vi "NEW RW Controls INI.vi"(1 "Filepath":path, 2 "Read (F)":bool, 7 "ControlArray In":T1(array[cluster]), 11 "Error In":errorcluster) -> (8 "ControlArray Out":T1(array[cluster]), 15 "Error Out":errorcluster)   [LabVIEW 2013]
uses:
  <vilib>/Utility/config.llb/Read Key (Double).vi
  <vilib>/Utility/config.llb/Write Key (Double).vi
  <vilib>/Utility/config.llb/NI_LVConfig.lvlib
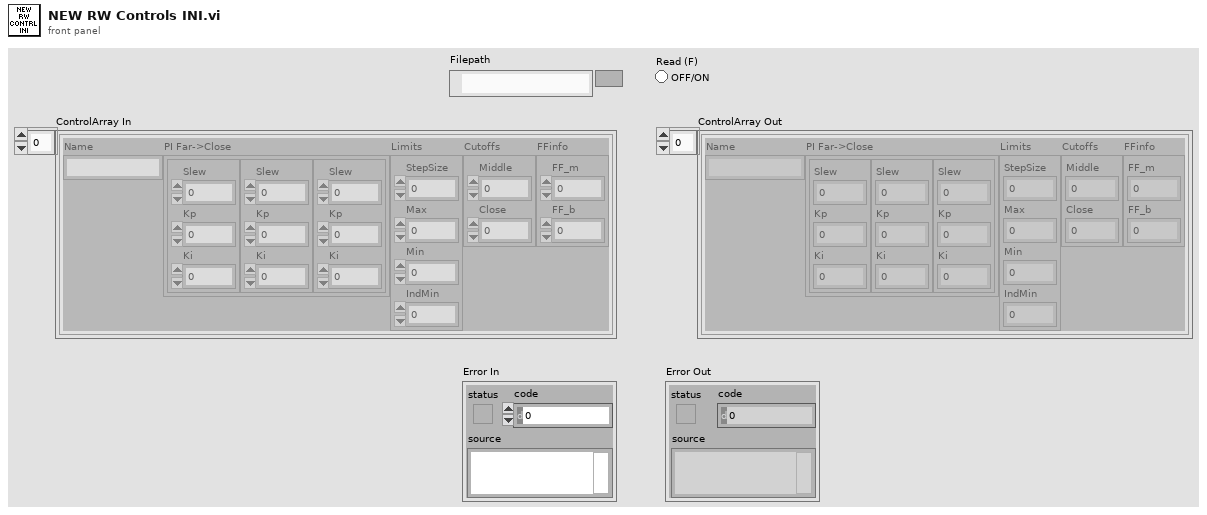
[diagram p1: front panel]
types:
  T1 = cluster{"Name":string, "PI Far->Close":cluster{"Slew":dbl, "Kp":dbl, "Ki":dbl}[], "Limits":cluster{"StepSize":dbl, "Max":dbl, "Min":dbl, "IndMin":dbl}, "Cutoffs":cluster{"Middle":dbl, "Close":dbl}, "FFinfo":cluster{"FF_m":dbl, "FF_b":dbl}}[]
  T2 = typedef "NI_LVConfig.lvlib/Config Data RefNum.ctl" = refnum<k1>
  T3 = cluster{"StepSize":dbl, "Max":dbl, "Min":dbl, "IndMin":dbl}
  T4 = cluster{"value":dbl, "value":dbl, "value":dbl, "value":dbl}
  T5 = cluster{"Name":string, "PI Far->Close":cluster{"Slew":dbl, "Kp":dbl, "Ki":dbl}[], "Limits":cluster{"StepSize":dbl, "Max":dbl, "Min":dbl, "IndMin":dbl}, "Cutoffs":cluster{"Middle":dbl, "Close":dbl}, "FFinfo":cluster{"FF_m":dbl, "FF_b":dbl}}
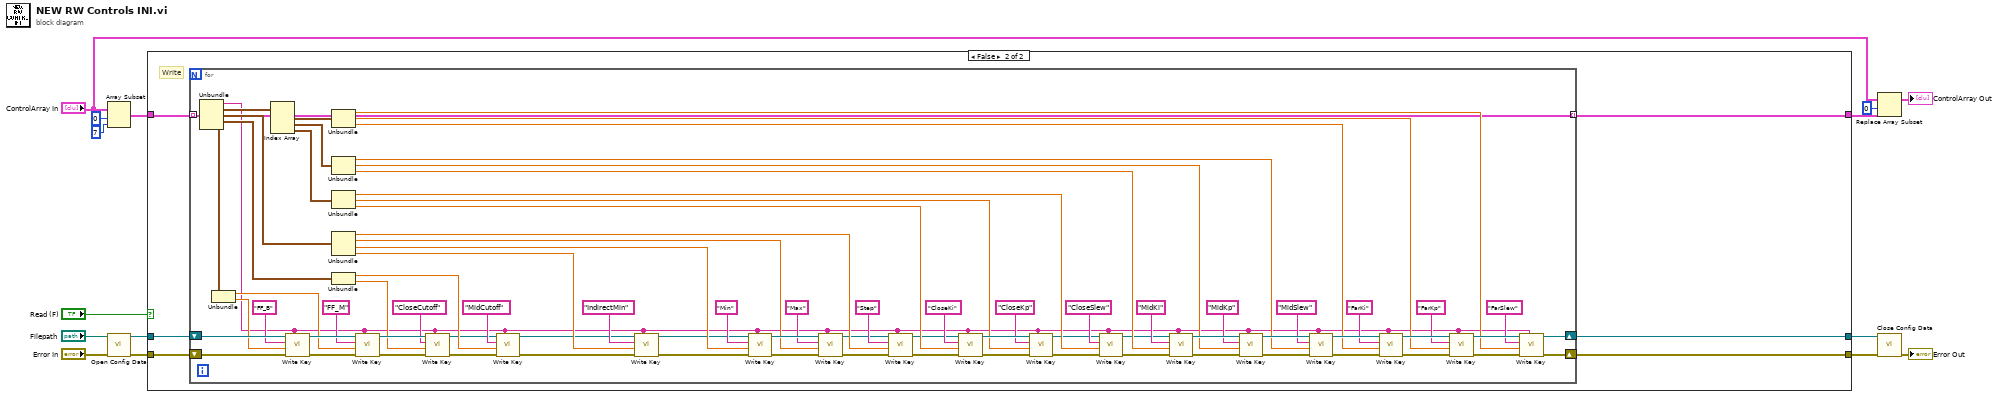
[diagram p0: block diagram]
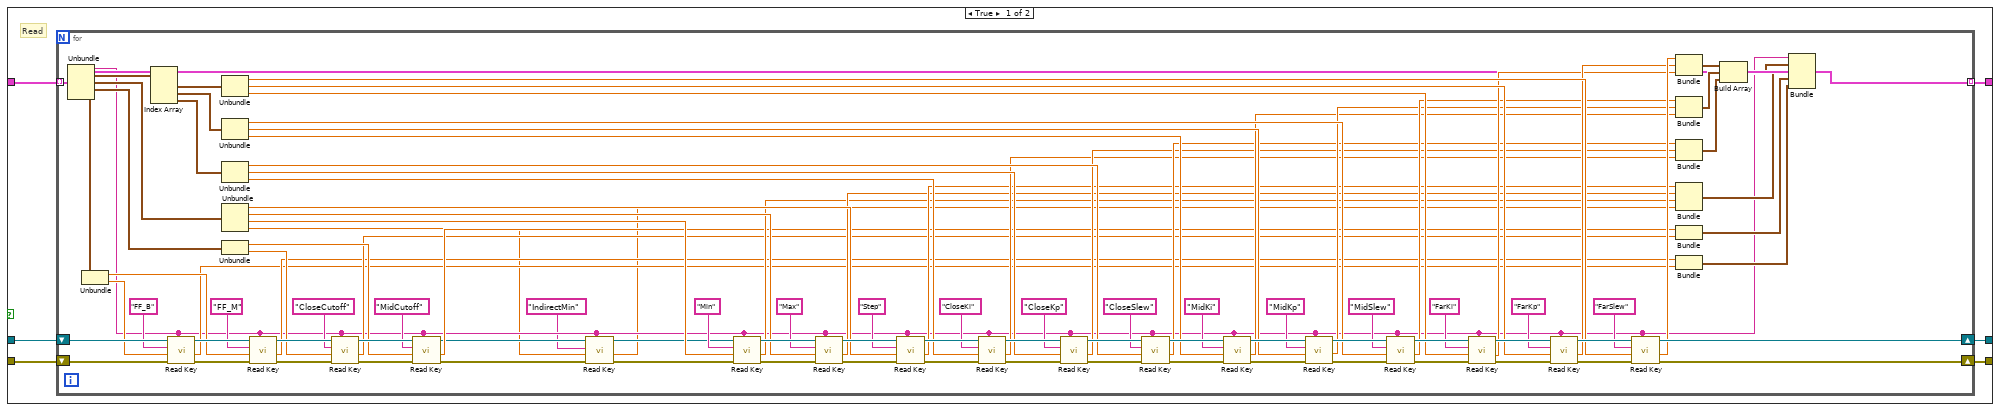
[diagram p2: hidden frame]
diagram:
  n1 = Array Subset(array="ControlArray In", index=0, length=7) -> (w1:T1)
  n2 = call <vilib>:"Open Config Data.vi"("error in (no error)"="Error In", "configuration file path"="Filepath") -> ("error out"=w11:errorcluster, "refnum"=w10:T2)  [unwired: 7 in, 1 out]
  n3 = case shown="False" "Read (F)" {
    tunnel: w11 -> [w17 w131]
    tunnel: w10 -> [w18 w130]
    tunnel: w1 -> [w21 w129]
    tunnel: [w20 w128] -> w9
    tunnel: [w19 w127] -> w8
    tunnel: [w16 w126] -> w5
    frame True {
      # "Read"
      n4 = for {
        tunnel: w21 -> [w35] mode=indexing
        shift-right: [w89] -> w19
        shift-left: w18 -> [w87]
        shift-right: [w90] -> w20
        shift-left: w17 -> [w88]
        tunnel: [w30] -> w16 mode=indexing
        n5 = Unbundle(w35) -> ("Name"=w28:string, "PI Far->Close"=w125:cluster{"Slew":dbl, "Kp":dbl, "Ki":dbl}[], "Limits"=w122:T3, "Cutoffs"=w123:cluster{"Middle":dbl, "Close":dbl}, "FFinfo"=w124:cluster{"FF_m":dbl, "FF_b":dbl})
        n6 = Unbundle(w124) -> ("FF_m"=w69:dbl, "FF_b"=w86:dbl)
        n7 = Index Array(array=w125) -> (element #1=w119:cluster{"Slew":dbl, "Kp":dbl, "Ki":dbl}, element #2=w120:cluster{"Slew":dbl, "Kp":dbl, "Ki":dbl}, element #3=w121:cluster{"Slew":dbl, "Kp":dbl, "Ki":dbl})  [unwired: 3 in]
        n8 = call-poly <vilib>:"Read Key.vi"("section"=w28, "error in (no error)"=w88, "default value"=w86, "key"="FF_B", "refnum"=w87) -> ("error out"=w117:errorcluster, "value"=w39:dbl, "refnum out"=w118:T2)  [unwired: 3 in, 1 out]
        n9 = Unbundle(w119) -> ("Slew"=w55:dbl, "Kp"=w56:dbl, "Ki"=w57:dbl)
        n10 = Unbundle(w120) -> ("Slew"=w58:dbl, "Kp"=w59:dbl, "Ki"=w60:dbl)
        n11 = Unbundle(w121) -> ("Slew"=w61:dbl, "Kp"=w62:dbl, "Ki"=w63:dbl)
        n12 = Unbundle(w122) -> ("StepSize"=w64:dbl, "Max"=w65:dbl, "Min"=w66:dbl, "IndMin"=w24:dbl)
        n13 = Unbundle(w123) -> ("Middle"=w67:dbl, "Close"=w68:dbl)
        n14 = call-poly <vilib>:"Read Key.vi"("section"=w28, "error in (no error)"=w117, "default value"=w69, "key"="FF_M", "refnum"=w118) -> ("error out"=w116:errorcluster, "value"=w40:dbl, "refnum out"=w115:T2)  [unwired: 3 in, 1 out]
        n15 = call-poly <vilib>:"Read Key.vi"("section"=w28, "error in (no error)"=w116, "default value"=w68, "key"="CloseCutoff", "refnum"=w115) -> ("error out"=w113:errorcluster, "value"=w41:dbl, "refnum out"=w114:T2)  [unwired: 3 in, 1 out]
        n16 = call-poly <vilib>:"Read Key.vi"("section"=w28, "error in (no error)"=w113, "default value"=w67, "key"="MidCutoff", "refnum"=w114) -> ("error out"=w26:errorcluster, "value"=w42:dbl, "refnum out"=w29:T2)  [unwired: 3 in, 1 out]
        n17 = call-poly <vilib>:"Read Key.vi"("section"=w28, "error in (no error)"=w26, "default value"=w24, "key"="IndirectMin", "refnum"=w29) -> ("error out"=w25:errorcluster, "value"=w23:dbl, "refnum out"=w27:T2)  [unwired: 3 in, 1 out]
        n18 = call-poly <vilib>:"Read Key.vi"("section"=w28, "error in (no error)"=w25, "default value"=w66, "key"="Min", "refnum"=w27) -> ("error out"=w112:errorcluster, "value"=w43:dbl, "refnum out"=w105:T2)  [unwired: 3 in, 1 out]
        n19 = call-poly <vilib>:"Read Key.vi"("section"=w28, "error in (no error)"=w112, "default value"=w65, "key"="Max", "refnum"=w105) -> ("error out"=w111:errorcluster, "value"=w44:dbl, "refnum out"=w104:T2)  [unwired: 3 in, 1 out]
        n20 = call-poly <vilib>:"Read Key.vi"("section"=w28, "error in (no error)"=w111, "default value"=w64, "key"="Step", "refnum"=w104) -> ("error out"=w110:errorcluster, "value"=w45:dbl, "refnum out"=w103:T2)  [unwired: 3 in, 1 out]
        n21 = call-poly <vilib>:"Read Key.vi"("section"=w28, "error in (no error)"=w110, "default value"=w63, "key"="CloseKi", "refnum"=w103) -> ("error out"=w109:errorcluster, "value"=w46:dbl, "refnum out"=w102:T2)  [unwired: 3 in, 1 out]
        n22 = call-poly <vilib>:"Read Key.vi"("section"=w28, "error in (no error)"=w109, "default value"=w62, "key"="CloseKp", "refnum"=w102) -> ("error out"=w108:errorcluster, "value"=w47:dbl, "refnum out"=w101:T2)  [unwired: 3 in, 1 out]
        n23 = call-poly <vilib>:"Read Key.vi"("section"=w28, "error in (no error)"=w108, "default value"=w61, "key"="CloseSlew", "refnum"=w101) -> ("error out"=w107:errorcluster, "value"=w48:dbl, "refnum out"=w100:T2)  [unwired: 3 in, 1 out]
        n24 = call-poly <vilib>:"Read Key.vi"("section"=w28, "error in (no error)"=w107, "default value"=w60, "key"="MidKi", "refnum"=w100) -> ("error out"=w106:errorcluster, "value"=w49:dbl, "refnum out"=w99:T2)  [unwired: 3 in, 1 out]
        n25 = call-poly <vilib>:"Read Key.vi"("section"=w28, "error in (no error)"=w106, "default value"=w59, "key"="MidKp", "refnum"=w99) -> ("error out"=w95:errorcluster, "value"=w50:dbl, "refnum out"=w98:T2)  [unwired: 3 in, 1 out]
        n26 = call-poly <vilib>:"Read Key.vi"("section"=w28, "error in (no error)"=w95, "default value"=w58, "key"="MidSlew", "refnum"=w98) -> ("error out"=w94:errorcluster, "value"=w51:dbl, "refnum out"=w97:T2)  [unwired: 3 in, 1 out]
        n27 = call-poly <vilib>:"Read Key.vi"("section"=w28, "error in (no error)"=w94, "default value"=w57, "key"="FarKi", "refnum"=w97) -> ("error out"=w93:errorcluster, "value"=w52:dbl, "refnum out"=w96:T2)  [unwired: 3 in, 1 out]
        n28 = call-poly <vilib>:"Read Key.vi"("section"=w28, "error in (no error)"=w93, "default value"=w56, "key"="FarKp", "refnum"=w96) -> ("error out"=w91:errorcluster, "value"=w53:dbl, "refnum out"=w92:T2)  [unwired: 3 in, 1 out]
        n29 = call-poly <vilib>:"Read Key.vi"("section"=w28, "error in (no error)"=w91, "default value"=w55, "key"="FarSlew", "refnum"=w92) -> ("error out"=w90:errorcluster, "value"=w54:dbl, "refnum out"=w89:T2)  [unwired: 3 in, 1 out]
        n30 = Bundle("value"=w54, "value"=w53, "value"=w52) -> (w38:cluster{"value":dbl, "value":dbl, "value":dbl})  [unwired: 1 in]
        n31 = Bundle("value"=w51, "value"=w50, "value"=w49) -> (w37:cluster{"value":dbl, "value":dbl, "value":dbl})  [unwired: 1 in]
        n32 = Bundle("value"=w48, "value"=w47, "value"=w46) -> (w36:cluster{"value":dbl, "value":dbl, "value":dbl})  [unwired: 1 in]
        n33 = Bundle("value"=w45, "value"=w44, "value"=w43, "value"=w23) -> (w33:T4)  [unwired: 1 in]
        n34 = Bundle("value"=w42, "value"=w41) -> (w32:cluster{"value":dbl, "value":dbl})  [unwired: 1 in]
        n35 = Bundle("value"=w40, "value"=w39) -> (w31:cluster{"value":dbl, "value":dbl})  [unwired: 1 in]
        n36 = Build Array(w38, w37, w36) -> (w34:cluster{"value":dbl, "value":dbl, "value":dbl}[])
        n37 = Bundle(cluster=w35, "Name"=w28, "PI Far->Close"=w34, "Limits"=w33, "Cutoffs"=w32, "FFinfo"=w31) -> (w30:T5)
      }
    }
    frame False {
      # "Write"
      n38 = for {
        tunnel: w129 -> [w139] mode=indexing
        shift-right: [w202] -> w127
        shift-left: w130 -> [w195]
        shift-right: [w203] -> w128
        shift-left: w131 -> [w192]
        tunnel: [w139] -> w126 mode=indexing
        n39 = Unbundle(w139) -> ("Name"=w132:string, "PI Far->Close"=w210:cluster{"Slew":dbl, "Kp":dbl, "Ki":dbl}[], "Limits"=w207:T3, "Cutoffs"=w208:cluster{"Middle":dbl, "Close":dbl}, "FFinfo"=w209:cluster{"FF_m":dbl, "FF_b":dbl})
        n40 = Unbundle(w209) -> ("FF_m"=w189:dbl, "FF_b"=w193:dbl)
        n41 = Index Array(array=w210) -> (element #1=w204:cluster{"Slew":dbl, "Kp":dbl, "Ki":dbl}, element #2=w205:cluster{"Slew":dbl, "Kp":dbl, "Ki":dbl}, element #3=w206:cluster{"Slew":dbl, "Kp":dbl, "Ki":dbl})  [unwired: 3 in]
        n42 = call-poly <vilib>:"Write Key.vi"("section"=w132, "error in (no error)"=w192, "value"=w193, "key"="FF_B", "refnum"=w195) -> ("error out"=w190:errorcluster, "refnum out"=w191:T2)  [unwired: 4 in, 1 out]
        n43 = Unbundle(w204) -> ("Slew"=w141:dbl, "Kp"=w142:dbl, "Ki"=w144:dbl)
        n44 = Unbundle(w205) -> ("Slew"=w147:dbl, "Kp"=w151:dbl, "Ki"=w156:dbl)
        n45 = Unbundle(w206) -> ("Slew"=w160:dbl, "Kp"=w163:dbl, "Ki"=w168:dbl)
        n46 = Unbundle(w207) -> ("StepSize"=w172:dbl, "Max"=w175:dbl, "Min"=w179:dbl, "IndMin"=w137:dbl)
        n47 = Unbundle(w208) -> ("Middle"=w182:dbl, "Close"=w186:dbl)
        n48 = call-poly <vilib>:"Write Key.vi"("section"=w132, "error in (no error)"=w190, "value"=w189, "key"="FF_M", "refnum"=w191) -> ("error out"=w185:errorcluster, "refnum out"=w187:T2)  [unwired: 4 in, 1 out]
        n49 = call-poly <vilib>:"Write Key.vi"("section"=w132, "error in (no error)"=w185, "value"=w186, "key"="CloseCutoff", "refnum"=w187) -> ("error out"=w183:errorcluster, "refnum out"=w180:T2)  [unwired: 4 in, 1 out]
        n50 = call-poly <vilib>:"Write Key.vi"("section"=w132, "error in (no error)"=w183, "value"=w182, "key"="MidCutoff", "refnum"=w180) -> ("error out"=w135:errorcluster, "refnum out"=w136:T2)  [unwired: 4 in, 1 out]
        n51 = call-poly <vilib>:"Write Key.vi"("section"=w132, "error in (no error)"=w135, "value"=w137, "key"="IndirectMin", "refnum"=w136) -> ("error out"=w134:errorcluster, "refnum out"=w133:T2)  [unwired: 4 in, 1 out]
        n52 = call-poly <vilib>:"Write Key.vi"("section"=w132, "error in (no error)"=w134, "value"=w179, "key"="Min", "refnum"=w133) -> ("error out"=w174:errorcluster, "refnum out"=w177:T2)  [unwired: 4 in, 1 out]
        n53 = call-poly <vilib>:"Write Key.vi"("section"=w132, "error in (no error)"=w174, "value"=w175, "key"="Max", "refnum"=w177) -> ("error out"=w171:errorcluster, "refnum out"=w170:T2)  [unwired: 4 in, 1 out]
        n54 = call-poly <vilib>:"Write Key.vi"("section"=w132, "error in (no error)"=w171, "value"=w172, "key"="Step", "refnum"=w170) -> ("error out"=w169:errorcluster, "refnum out"=w166:T2)  [unwired: 4 in, 1 out]
        n55 = call-poly <vilib>:"Write Key.vi"("section"=w132, "error in (no error)"=w169, "value"=w168, "key"="CloseKi", "refnum"=w166) -> ("error out"=w162:errorcluster, "refnum out"=w165:T2)  [unwired: 4 in, 1 out]
        n56 = call-poly <vilib>:"Write Key.vi"("section"=w132, "error in (no error)"=w162, "value"=w163, "key"="CloseKp", "refnum"=w165) -> ("error out"=w161:errorcluster, "refnum out"=w158:T2)  [unwired: 4 in, 1 out]
        n57 = call-poly <vilib>:"Write Key.vi"("section"=w132, "error in (no error)"=w161, "value"=w160, "key"="CloseSlew", "refnum"=w158) -> ("error out"=w157:errorcluster, "refnum out"=w154:T2)  [unwired: 4 in, 1 out]
        n58 = call-poly <vilib>:"Write Key.vi"("section"=w132, "error in (no error)"=w157, "value"=w156, "key"="MidKi", "refnum"=w154) -> ("error out"=w150:errorcluster, "refnum out"=w153:T2)  [unwired: 4 in, 1 out]
        n59 = call-poly <vilib>:"Write Key.vi"("section"=w132, "error in (no error)"=w150, "value"=w151, "key"="MidKp", "refnum"=w153) -> ("error out"=w146:errorcluster, "refnum out"=w149:T2)  [unwired: 4 in, 1 out]
        n60 = call-poly <vilib>:"Write Key.vi"("section"=w132, "error in (no error)"=w146, "value"=w147, "key"="MidSlew", "refnum"=w149) -> ("error out"=w199:errorcluster, "refnum out"=w198:T2)  [unwired: 4 in, 1 out]
        n61 = call-poly <vilib>:"Write Key.vi"("section"=w132, "error in (no error)"=w199, "value"=w144, "key"="FarKi", "refnum"=w198) -> ("error out"=w196:errorcluster, "refnum out"=w197:T2)  [unwired: 4 in, 1 out]
        n62 = call-poly <vilib>:"Write Key.vi"("section"=w132, "error in (no error)"=w196, "value"=w142, "key"="FarKp", "refnum"=w197) -> ("error out"=w201:errorcluster, "refnum out"=w200:T2)  [unwired: 4 in, 1 out]
        n63 = call-poly <vilib>:"Write Key.vi"("section"=w132, "error in (no error)"=w201, "value"=w141, "key"="FarSlew", "refnum"=w200) -> ("error out"=w203:errorcluster, "refnum out"=w202:T2)  [unwired: 4 in, 1 out]
      }
    }
  }
  n64 = Replace Array Subset(array="ControlArray In", new element=w5, index=0) -> (→"ControlArray Out":T1)
  n65 = call <vilib>:"Close Config Data.vi"("error in (no error)"=w9, "refnum"=w8) -> ("error out"=→"Error Out":errorcluster)  [unwired: 8 in, 1 out]
